vi "myAppLauncher.vi"() -> ()   [LabVIEW 2013]
uses:
  ApplicationExample/Controller/MyAppController.lvclass
  View/base/VIEW.lvclass
  CONTROLLER.lvclass
  ApplicationExample/View/myAppView.lvclass
panel:
  in  "FrameworkDefaults":bool
  out "error out":errorcluster
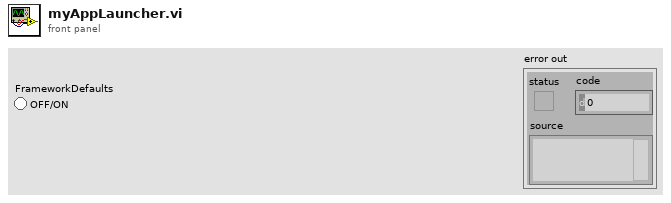
[diagram p1: front panel]
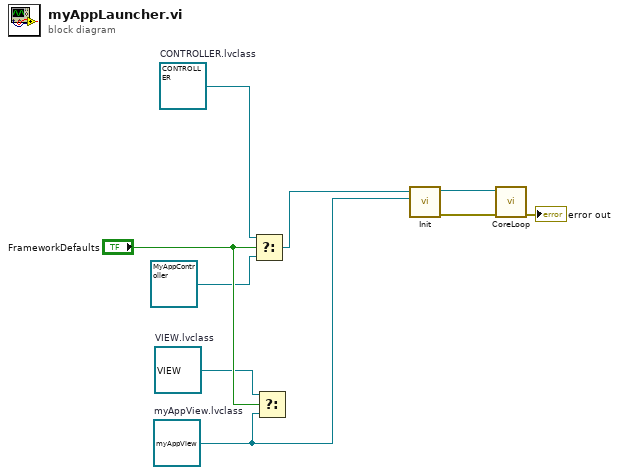
[diagram p0: block diagram]
diagram:
  w4 = refnum<class "myAppView.lvclass"> refnum  # myAppView.lvclass
  w3 = refnum<class "CONTROLLER.lvclass"> refnum  # CONTROLLER.lvclass
  w5 = refnum<class "VIEW.lvclass"> refnum  # VIEW.lvclass
  n1 = Select(t=w3, s="FrameworkDefaults", f=refnum<class "MyAppController.lvclass"> refnum ("MyAppController.lvclass")) -> (s? t:f=w1:refnum<class "CONTROLLER.lvclass">)
  n2 = Select(t=w5, s="FrameworkDefaults", f=w4) -> ()  [unwired: 1 out]
  n3 = call-dynamic "Init.vi"("VIEW"=w4, "CONTROLLER in"=w1) -> ("error out"=w7:errorcluster, "CONTROLLER out"=w9:refnum<class "CONTROLLER.lvclass">)  [unwired: 8 in]
  n4 = call-dynamic "CoreLoop.vi"("error in (no error)"=w7, "CONTROLLER in"=w9) -> ("error out"=→"error out":errorcluster)  [unwired: 8 in, 1 out]
